vi "Create Child Element.vi"(8 "error in (no error)":errorcluster, 9 "Value (\"\")":string, 10 "Name":string="testsuite", 11 "Node in":refnum<k20>) -> (0 "error out":errorcluster, 2 "Child Element":refnum<k20>, 3 "Node out":refnum<k20>)   [LabVIEW 2013, in "JUnit XML.lvlib"]
doc: "Creates a new child element with the specified name and value under the provided node and returns the created element. The caller is responsible for cleaning up references.\n\nThe provided node can either be another element or the document."
uses:
  JUnit XML.lvlib
  <vilib>/xml/Close Reference(Node).vi
  <resource>/objmgr/DOMUserDefRef.rc
  <vilib>/xml/NI_XML.lvlib
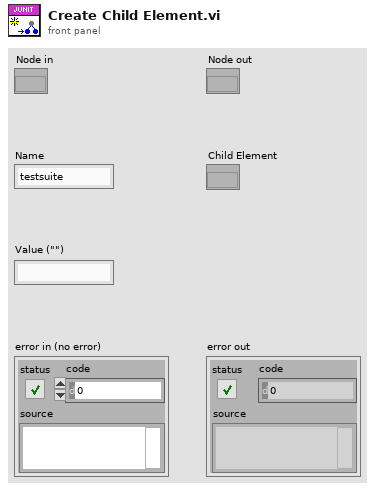
[diagram p1: front panel]
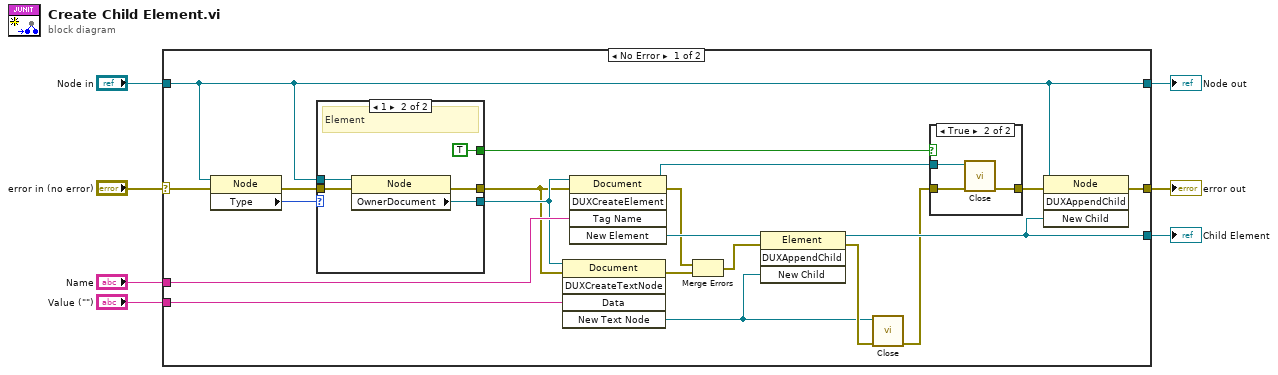
[diagram p0: block diagram]
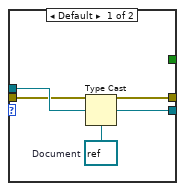
[diagram p3: hidden frame]
diagram:
  n1 = case shown="No Error" "error in (no error)" {
    selector: "error in (no error)" -> [w11 w42]
    tunnel: [w16 _] -> w7
    tunnel: "Node in" -> [w12 w41]
    tunnel: [w12 w41] -> w5
    tunnel: "Name" -> [w27 _]
    tunnel: [w26 w42] -> w3
    tunnel: "Value (\"\")" -> [w25 _]
    frame No Error {
      n2 = property class="Node"(reference=w12, error in=w11) -> (error out=w10:errorcluster, "Type"=w9:i32)  [unwired: 1 out]
      n3 = case shown="1" w9 {
        tunnel: w10 -> [w32 w40]
        tunnel: [w33 w39] -> w23
        tunnel: [w32 w38] -> w22
        tunnel: w12 -> [w35 w37]
        tunnel: [_ TRUE] -> w8
        frame Default {
          w34 = refnum<k20> refnum  # Document
          n4 = Type Cast(type=w34, x=w35) -> (*(type *) &x=w33:refnum<k20>)
        }
        frame 1 {
          # "Element"
          n5 = property class="Node"(reference=w37, error in=w40) -> (error out=w38:errorcluster, "OwnerDocument"=w39:refnum<k20>)  [unwired: 1 out]
        }
      }
      n6 = invoke class="Document" method="DUXCreateTextNode"(reference=w23, error in=w22, "Data"=w25) -> (error out=w20:errorcluster, "New Text Node"=w17:refnum<k20>)  [unwired: 2 in, 3 out]
      n7 = invoke class="Document" method="DUXCreateElement"(reference=w23, error in=w22, "Tag Name"=w27) -> (reference out=w13:refnum<k20>, error out=w21:errorcluster, "New Element"=w24:refnum<k20>)  [unwired: 2 in, 2 out]
      n8 = Merge Errors(w21, w20) -> (w19:errorcluster)
      n9 = invoke class="Element" method="DUXAppendChild"(reference=w24, error in=w19, "New Child"=w17) -> (reference out=w16:refnum<k20>, error out=w18:errorcluster)  [unwired: 1 in, 2 out]
      n10 = call-poly <vilib>:"Close.vi"("error in (no error)"=w18, "node"=w17) -> ("error out"=w14:errorcluster)  [unwired: 7 in]
      n11 = case shown="True" w8 {
        tunnel: [w28 w31] -> w15
        tunnel: w14 -> [w28 w30]
        tunnel: w13 -> [_ w29]
        frame False {
        }
        frame True {
          n12 = call-poly <vilib>:"Close.vi"("error in (no error)"=w30, "node"=w29) -> ("error out"=w31:errorcluster)  [unwired: 7 in]
        }
      }
      n13 = invoke class="Node" method="DUXAppendChild"(reference=w12, error in=w15, "New Child"=w16) -> (error out=w26:errorcluster)  [unwired: 1 in, 3 out]
    }
    frame Error {
    }
  }
  "Node out" <- w5
  "Child Element" <- w7
  "error out" <- w3
